vi "Pane Check Pos.vi"(8 "Control Coordinates":T1, 11 "Pane Coordinates":T1) -> (0 "Left?":bool, 1 "Bottom?":bool, 2 "Right?":bool, 3 "Top?":bool)   [LabVIEW 2018]
uses:
  Pane Object.lvclass/Object Coordinates.ctl
  Pane Object.lvclass/Pane Object Position.lvclass
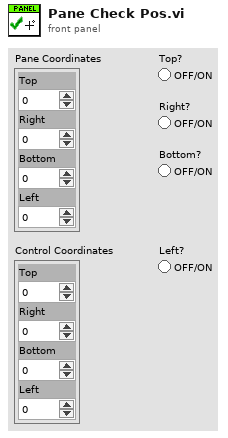
[diagram p1: front panel]
types:
  T1 = typedef "Pane Object Position.lvclass/Object Coordinates.ctl" = cluster{"Top":i32, "Right":i32, "Bottom":i32, "Left":i32}
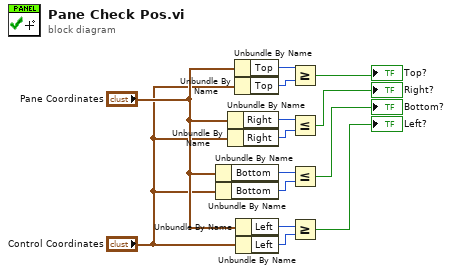
[diagram p0: block diagram]
diagram:
  n1 = Unbundle By Name("Pane Coordinates") -> ("Bottom"=w7:i32)
  n2 = Unbundle By Name("Control Coordinates") -> ("Bottom"=w8:i32)
  n3 = Unbundle By Name("Pane Coordinates") -> ("Right"=w5:i32)
  n4 = Unbundle By Name("Control Coordinates") -> ("Right"=w6:i32)
  n5 = Unbundle By Name("Pane Coordinates") -> ("Top"=w3:i32)
  n6 = Unbundle By Name("Control Coordinates") -> ("Top"=w4:i32)
  n7 = Unbundle By Name("Pane Coordinates") -> ("Left"=w9:i32)
  n8 = Unbundle By Name("Control Coordinates") -> ("Left"=w10:i32)
  n9 = Greater Or Equal?(x=w3, y=w4) -> (x >= y?=→"Top?":bool)
  n10 = Less Or Equal?(x=w5, y=w6) -> (x <= y?=→"Right?":bool)
  n11 = Less Or Equal?(x=w7, y=w8) -> (x <= y?=→"Bottom?":bool)
  n12 = Greater Or Equal?(x=w9, y=w10) -> (x >= y?=→"Left?":bool)
